vi "Process.vi"(8 "error in (no error)":errorcluster, 9 "Galvo.lvclass":refnum<class "Galvo.lvclass">, 10 "DAQ Class.lvclass":refnum<class "DAQ Class.lvclass">, 11 "Intensity Processing in":refnum<class "Intensity Processing.lvclass">) -> (0 "error out":errorcluster, 3 "Intensity Processing out":refnum<class "Intensity Processing.lvclass">)   [LabVIEW 2015, in "Intensity Processing.lvclass"]
uses:
  Intensity Processing.lvclass
  DAQ/DAQ Class.lvclass
  Galvo/Galvo.lvclass
  En Face States.ctl
  DAQ/DAQ Control Functional Global States.ctl
  Intensity Processing.lvclass/Intensity Processing.ctl
  <vilib>/Analysis/4window.llb/Hanning Window (DBL).vi
  <vilib>/Analysis/2dsp.llb/Real FFT.vi
  <vilib>/Analysis/4window.llb/AllCosWindow (DBL).vi
  Processing.lvclass
  Filter/Filter.lvclass
  <vilib>/Analysis/NI_AALPro.lvlib
panel:
  out "Stop Trim":dbl
  out "Start Trim":dbl
  out "Save Data":bool
  out "Save File Refnum":refnum<file>
  out "B-Scans Per Transfer":u32
  out "Points Per A-Scan":u32
  out "A-Scans Per B-Scan":u32
  out "Number of B-Scans":u32
  out "Background Noise":dbl[](array[numeric])
  out "Gain":dbl
  out "Log?":bool=TRUE
  out "Intensity Graph":sgl[][](graph)
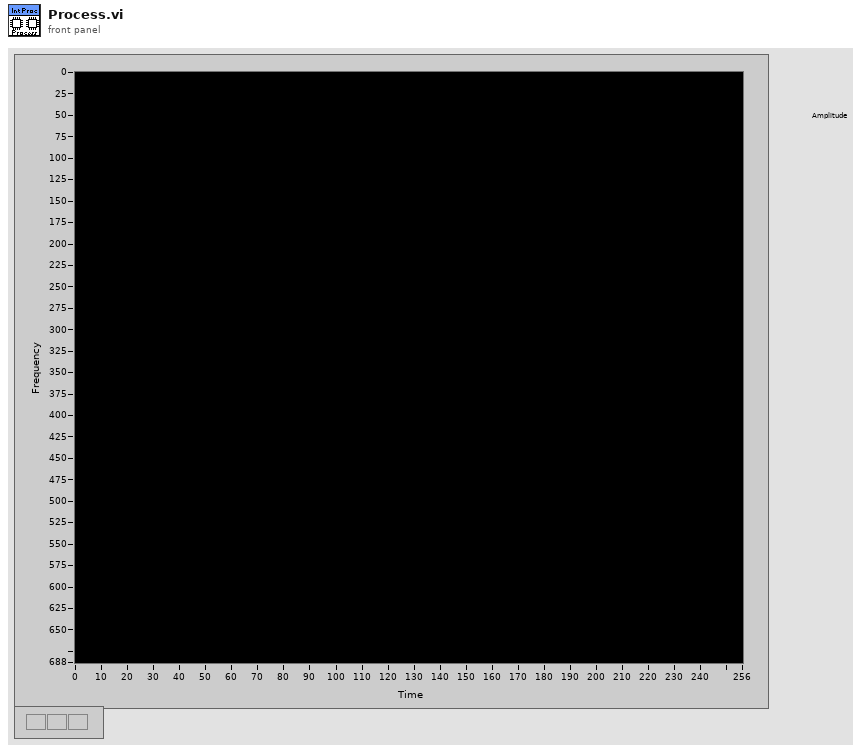
[diagram p1: front panel]
types:
  T1 = typedef "En Face States.ctl" = enum16{"Reset", "Update", "Get EnFace"}
  T2 = typedef "DAQ Class.lvclass/DAQ Parameters.ctl" = cluster{"Points Per A-Scan":u32, "A-Scans Per B-Scan":u32, "Number of B-Scans":u32, "B-Scans Per Transfer":u32, "Trigger Voltage":sgl, "Trigger Source":T3, "Trigger Slope":T4, "Channel":T5, "Clock":T6, "Bits per Sample":dbl, "Range":dbl, "Start Trim":u32, "Stop Trim":u32}
  T3 = typedef "DAQ Class.lvclass/Trigger Source.ctl" = enum16{"External", "Channel A", "Channel B"}
  T4 = typedef "DAQ Class.lvclass/Trigger Slope.ctl" = enum16{"Rising", "Falling"}
  T5 = typedef "OCT DAQ Channel Data Type.ctl" = enum16{"Channel 1", "Channel 2", "Channel 1 and 2"}
  T6 = typedef "DAQ Class.lvclass/Clock Control.ctl" = enum16{"Internal Clock", "External Clock"}
  T7 = enum16{"open", "replace", "create", "open or create", "replace or create", "replace or create with confirmation"}
  T8 = typedef "Galvo.lvclass/Scanning Cluster.ctl" = cluster{"Fast Axis Offset":sgl, "Slow Axis Offset":sgl, "Slow Axis Amp":sgl, "Fast Axis Amp":sgl, "Scan Pattern":enum16{"Raster", "Triangle Raster", "Sinusoid Raster"}}
  T9 = typedef "DAQ Control Functional Global States.ctl" = enum16{"Status", "Set Processing Finished", "Reset", "Clear", "Set DAQ Finished"}
  T10 = typedef "LVCursorListTypeDef.ctl" = cluster{"Name":string, "Color":u32, "Style":u8, "Point Style":u8, "Name Visible":bool, "Allow Drag":bool, "Cursor Mode":u32, "Plot":i32, "Index":i32, "Position":cluster{"X":dbl, "Y":dbl}, "X Scale":u32, "Y Scale":u32, "Watch Plots":i32[], "Watch All Plots":bool, "Plot Area":i32, "Label Offset":cluster{"X":dbl, "Y":dbl}}[]
  T11 = cluster{"Name":string, "Color":u32, "Style":u8, "Point Style":u8, "Name Visible":bool, "Allow Drag":bool, "Cursor Mode":u32, "Plot":i32, "Index":i32, "Position":cluster{"X":dbl, "Y":dbl}, "X Scale":u32, "Y Scale":u32, "Watch Plots":i32[], "Watch All Plots":bool, "Plot Area":i32, "Label Offset":cluster{"X":dbl, "Y":dbl}}
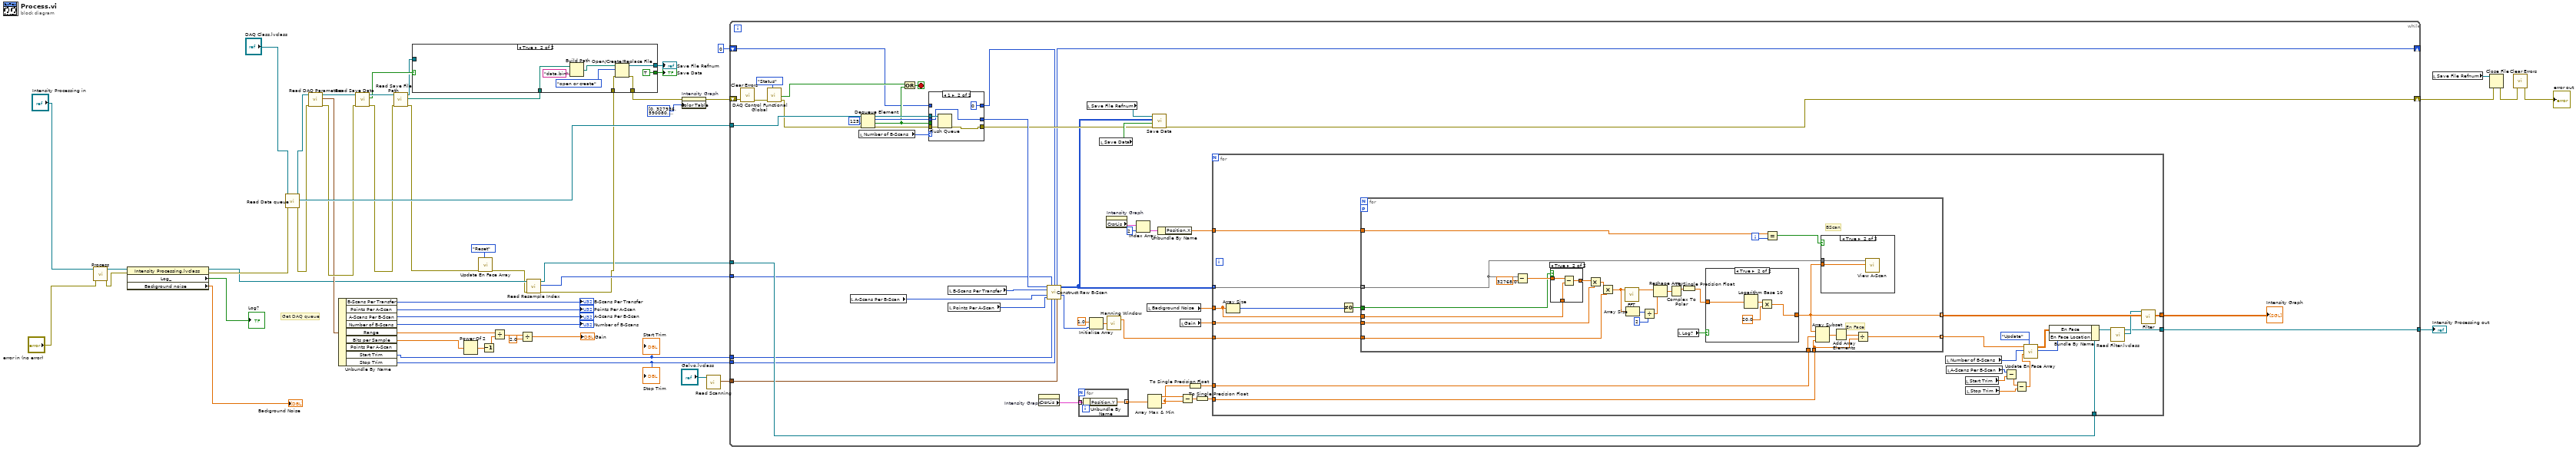
[diagram p0: block diagram]
diagram:
  # "Get DAQ queue"
  n1 = call-parent "Process.vi"("error in (no error)"="error in (no error)", "Processing in"="Intensity Processing in") -> ("error out"=w36:errorcluster, "Processing out"=w38:refnum<class "Intensity Processing.lvclass">)  [unwired: 8 in]
  n2 = property class="Intensity Processing.lvclass"(reference=w38, error in=w36) -> (reference out=w12:refnum<class "Intensity Processing.lvclass">, error out=w35:errorcluster, "Log_"=→"Log?":bool, "Background noise"=→"Background Noise":dbl[])
  n3 = call-dynamic "Read Data queue.vi"("error in (no error)"=w35, "DAQ Class in"="DAQ Class.lvclass") -> ("error out"=w50:errorcluster, "Data queue"=w51:refnum<queue>, "DAQ Class out"=w49:refnum<class "DAQ Class.lvclass">)  [unwired: 7 in]
  n4 = call-dynamic "Read DAQ Parameters.vi"("error in (no error)"=w50, "DAQ Class in"=w49) -> ("error out"=w32:errorcluster, "DAQ Parameters"=w26:T2, "DAQ Class out"=w34:refnum<class "DAQ Class.lvclass">)  [unwired: 7 in]
  n5 = Unbundle By Name(w26) -> ("B-Scans Per Transfer"=→"B-Scans Per Transfer":u32, "Points Per A-Scan"=→"Points Per A-Scan":u32, "A-Scans Per B-Scan"=→"A-Scans Per B-Scan":u32, "Number of B-Scans"=→"Number of B-Scans":u32, "Range"=w46:dbl, "Bits per Sample"=w47:dbl, "Start Trim"=w5:u32, "Stop Trim"=w6:u32)  [unwired: 1 out]
  "Start Trim" <- w5
  "Stop Trim" <- w6
  n6 = call-dynamic "Read Save Data.vi"("error in (no error)"=w32, "DAQ Class in"=w34) -> ("error out"=w33:errorcluster, "Save Data"=w30:bool, "DAQ Class out"=w31:refnum<class "DAQ Class.lvclass">)  [unwired: 7 in]
  n7 = call-dynamic "Read Save File Path.vi"("error in (no error)"=w33, "DAQ Class in"=w31) -> ("error out"=w17:errorcluster, "Save File Path"=w29:path, "DAQ Class out"=w25:refnum<class "DAQ Class.lvclass">)  [unwired: 7 in]
  n8 = Power Of 2(x=w47) -> (2^x=w48:dbl)
  n9 = call "Update En Face Array.vi"("State"=En_Face_States."Reset", "Error In"=w17) -> ("Error Out"=w9:errorcluster)  [unwired: 7 in, 2 out]
  n10 = Decrement(x=w48) -> (x-1=w45:dbl)
  n11 = Divide(x=w46, y=w45) -> (x/y=w24:dbl)
  n12 = Divide(x=w24, y=2.0) -> (x/y=→"Gain":dbl)
  n13 = call-dynamic "Read Resample Index.vi"("error in (no error)"=w9, "Processing in"=w12) -> ("error out"=w10:errorcluster, "Resample Index"=w11:i32[], "Processing out"=w8:refnum<class "Intensity Processing.lvclass">)  [unwired: 7 in]
  n14 = case shown="True" w30 {
    selector: w30 -> [w53 _]
    tunnel: w10 -> [w54 w62]
    tunnel: [w54 w61] -> w27
    tunnel: [_ w60] -> w15
    tunnel: [w53 TRUE] -> w14
    tunnel: w29 -> [_ w58]
    tunnel: w25 -> [_ _]
    frame False {
    }
    frame True {
      n15 = Build Path(base path=w58, name or relative path="data.bin") -> (appended path=w57:path)
      n16 = Open/Create/Replace File(file path (use dialog)=w57, error in=w62, operation (0:open)=T7."open or create") -> (refnum out=w60:refnum<file>, error out=w61:errorcluster)  [unwired: 3 in, 1 out]
    }
  }
  "Save File Refnum" <- w15
  "Save Data" <- w14
  n17 = property on="Intensity Graph" class="IntGraph (strict)"(error in=w27, "Color Table"=u32[] [0, 327936, 590080, 852224, 983296, 1114624, 1180160, 1311232, 1442304, 1573632, 1704704, 1770240, 1901312, 1966848, 2098176, 2163712, 2294784, 2491392, 2557184, 2688256, 2753792, 2884864, 2950656, 3081728, 3147264, 3344129, 3475457, 3540993, 3672321, 3738113, 3869185, 3934977, 4066305, 4197633, 4328961, 4394497, 4460289, 4591617, 4657409, 4788481, 4854273, 4985601, 5116929, 5248257, 5314049, 5379841, 5511169, 5576961, 5708033, 5773825, 5905153, 6036482, 6167810, 6233346, 6299138, 6430466, 6496258, 6562050, 6693634, 6759426, 6890754, 7022082, 7087874, 7153666, 7284994, 7350786, 7482114, 7547906, 7613698, 7745026, 7876354, 8007682, 8073474, 8139522, 8205314, 8336642, 8467970, 8533763, 8599555, 8665347, 8731139, 8862467, 8993795, 9059587, 9125380, 9191428, 9257220, 9388548, 9454340, 9520132, 9585924, 9717253, 9848837, 9914629, 9980165, 10045957, 10177541, 10243334, 10309126, 10375174, 10440966, 10572294, 10703623, 10769416, 10835208, 10901256, 10967049, 11033097, 11033609, 11099401, 11165450, 11231242, 11231754, 11297547, 11363339, 11429131, 11495180, 11495692, 11561740, 11693069, 11758861, 11759373, 11825165, 11891214, 11957006, 12022799, 12023311, 12089103, 12220944, 12286736, 12286736, 12352529, 12418577, 12484370, 12550162, 12615954, 12681747, 12747796, 12813588, 12813845, 12879894, 12945686, 13077015, 13142808, 13143064, 13208856, 13274905, 13340697, 13340953, 13472282, 13538075, 13604379, 13670172, 13735964, 13801757, 13867550, 13933343, 13999392, 13999648, 14065441, 14131234, 14197027, 14197541, 14263334, 14329383, 14395176, 14460969, 14592553, 14658346, 14724139, 14789932, 14790189, 14856238, 14922287, 14988080, 15053873, 15054130, 15119923, 15185972, 15251765, 15317559, 15383353, 15449146, 15449660, 15515454, 15515968, 15516226, 15582021, 15582278, 15582536, 15648587, 15648844, 15714639, 15714897, 15715155, 15780949, 15781463, 15847256, 15847770, 15848028, 15913823, 15914081, 15979875, 15980133, 15980391, 16046441, 16046444, 16046703, 16046705, 16112500, 16113015, 16113274, 16113277, 16179072, 16179330, 16179588, 16245384, 16245387, 16245389, 16245648, 16311443, 16376982, 16377241, 16377499, 16443294, 16443553, 16443555, 16443815, 16509866, 16510124, 16510127, 16575923, 16575924, 16576182, 16576441, 16576443, 16576702, 16576705, 16576963, 16577222, 16577224, 16577482, 16577485, 16577743, 16577745, 16578004, 16578262, 16578264, 16578523, 16578782, 16579040, 16579299, 16579301, 16579303, 16579562, 16579821]) -> (error out=w28:errorcluster)  [unwired: 1 in, 1 out]
  n18 = call-dynamic "Read Scanning.vi"("Galvo in"="Galvo.lvclass") -> ("Scanning Parameters"=w3:T8)  [unwired: 8 in, 2 out]
  n19 = while {
    tunnel: w51 -> [w101]
    shift-right: [w79] -> w43
    shift-left: w28 -> [w111]
    tunnel: w11 -> [w67]
    tunnel: w8 -> [w71]
    shift-right: [w70] -> _
    shift-left: 0 -> [w69]
    tunnel: w6 -> [w66]
    tunnel: w5 -> [w65]
    tunnel: w3 -> [w64]
    tunnel: [w63] -> w1
    stop <- w104 stop-if-true
    n20 = call <vilib>:"Clear Errors.vi"("error in (no error)"=w111) -> ("error out"=w110:errorcluster)  [unwired: 5 in, 1 out]
    n21 = call "DAQ Control Functional Global.vi"("State"=DAQ_Control_Functional_Global_States."Status", "Error In"=w110) -> ("Error Out"=w100:errorcluster, "Reset?"=w102:bool)  [unwired: 6 in, 2 out]
    n22 = local read "A-Scans Per B-Scan"() -> (w85:u32)
    n23 = local read "Number of B-Scans"() -> (w86:u32)
    n24 = Dequeue Element(queue=w101, timeout in ms (-1)=125, error in (no error)=w100) -> (queue out=w97:refnum<queue>, element=w98:u16[], timed out?=w94:bool, error out=w96:errorcluster)
    n25 = Or(x=w102, y=w94) -> (x .or. y?=w104:bool)
    n26 = case shown="1" w86 {
      tunnel: w98 -> [w177 w179]
      tunnel: w97 -> [_ w181]
      tunnel: [w177 w179] -> w89
      tunnel: w94 -> [_ _]
      tunnel: w96 -> [w176 w182]
      tunnel: [w176 w180] -> w80
      tunnel: w69 -> [w175 _]
      tunnel: [w175 u32 0 ("B-Scan Processed Out")] -> w68
      frame 0, Default {
      }
      frame 1 {
        n27 = Flush Queue(queue=w181, error in (no error)=w182) -> (error out=w180:errorcluster)  [unwired: 2 out]
      }
    }
    n28 = local read "B-Scans Per Transfer"() -> (w84:u32)
    n29 = local read "Points Per A-Scan"() -> (w83:u32)
    n30 = property on="Intensity Graph" class="IntGraph (strict)"() -> ("CrsrLis"=w106:T10)  [unwired: 2 in, 2 out]
    n31 = call "Construct Raw B-Scan.vi"("1D Raw Data In"=w89, "Resample Array"=w67, "B-Scan Processed In"=w68, "B-Scans Per Transfer"=w84, "A-Scans Per B-Scan"=w85, "Points Per A-Scan"=w83, "Start Trim"=w65, "Stop Trim"=w66, "Scanning Parameters"=w64) -> ("B-Scan Processed Out"=w70:u32, "B-Scan In"=w78:u16[][][], "A-Scan Size"=w74:i32)  [unwired: 4 in]
    n32 = for {
      tunnel: w106 -> [w184] mode=indexing
      tunnel: [w183] -> w105 mode=indexing
      n33 = Unbundle By Name(w184) -> ("Position.Y"=w183:dbl)
    }
    n34 = local read "Save File Refnum"() -> (w82:refnum<file>)
    n35 = Initialize Array(1.0 ("element"), w74) -> (w76:dbl[])
    n36 = local read "Save Data"() -> (w81:bool)
    n37 = property on="Intensity Graph" class="IntGraph (strict)"() -> ("CrsrLis"=w93:T10)  [unwired: 2 in, 2 out]
    n38 = call-poly <vilib>:"Hanning Window.vi"("X"=w76) -> ("Windowed X"=w75:dbl[])  [unwired: 1 out]
    n39 = Index Array(array=w93, index=2) -> (element=w91:T11)
    n40 = local read "Background Noise"() -> (w88:dbl[])
    n41 = Array Max & Min(array=w105) -> (max value=w109:dbl, min value=w107:dbl)  [unwired: 2 out]
    n42 = call "Save Data.vi"("error in (no error)"=w80, ">> Save Data? >>"=w81, "U16 Array"=w78, "Byte Stream File in"=w82) -> ("error out"=w79:errorcluster)  [unwired: 7 in]
    n43 = Unbundle By Name(w91) -> ("Position.X"=w90:dbl)
    n44 = local read "Gain"() -> (w87:dbl)
    n45 = Subtract(x=w109, y=w107) -> (x-y=w108:dbl)
    n46 = To Single Precision Float(number=w107) -> (single precision float=w72:sgl)
    n47 = To Single Precision Float(number=w108) -> (single precision float=w73:sgl)
    n48 = for {
      tunnel: w73 -> [w136]
      tunnel: w72 -> [w135]
      tunnel: w87 -> [w134]
      tunnel: [w125] -> w95
      tunnel: w90 -> [w131]
      tunnel: w78 -> [w122] mode=indexing
      tunnel: w88 -> [w130]
      tunnel: w75 -> [w129]
      tunnel: w71 -> [w116]
      tunnel: [w112] -> w63
      n49 = Array Size(array=w130) -> (size(s)=w133:i32)
      n50 = Not Equal To 0?(x=w133) -> (x != 0?=w132:bool)
      n51 = for {
        tunnel: w129 -> [w163]
        tunnel: [w139] -> w124 mode=indexing
        tunnel: w136 -> [w158]
        tunnel: w135 -> [w161]
        tunnel: [w138] -> w126 mode=indexing
        tunnel: w134 -> [w156]
        tunnel: w122 -> [w137] mode=indexing
        tunnel: w130 -> [w148]
        tunnel: w132 -> [w146]
        workers-P: _ -> [_]
        tunnel: w131 -> [w144]
        i -> [w145]
        # "BScan"
        # "En Face"
        n52 = Subtract(x=w137, y=32768.0) -> (x-y=w149:dbl[])
        n53 = case shown="True" w146 {
          tunnel: w149 -> [w166 w169]
          tunnel: w148 -> [_ w168]
          tunnel: [w166 w167] -> w147
          frame False {
          }
          frame True {
            n54 = Subtract(x=w169, y=w168) -> (x-y=w167:dbl[])
          }
        }
        n55 = Multiply(x=w147, y=w156) -> (x*y=w150:dbl[])
        n56 = Multiply(x=w150, y=w163) -> (x*y=w152:dbl[])
        n57 = call-poly <vilib>:"FFT.vi"("X"=w152) -> ("FFT {X}"=w162:cdb[])  [unwired: 9 in, 1 out]
        n58 = Array Size(array=w152) -> (size(s)=w155:i32)
        n59 = Divide(x=w155, y=2) -> (x/y=w153:dbl)
        n60 = Reshape Array(w162, w153) -> (w142:cdb[])
        n61 = Complex To Polar(r * e^(i*theta)=w142) -> (r=w141:dbl[])  [unwired: 1 out]
        n62 = local read "Log?"() -> (w157:bool)
        n63 = To Single Precision Float(number=w141) -> (single precision float=w140:sgl[])
        n64 = case shown="True" w157 {
          tunnel: w140 -> [w170 w174]
          tunnel: [w170 w171] -> w139
          frame False {
          }
          frame True {
            n65 = Logarithm Base 10(1:w174) -> (0:w173:sgl[])
            n66 = Multiply(x=w173, y=sgl 20.0 ("element")) -> (x*y=w171:sgl[])
          }
        }
        n67 = Equal?(x=w144, y=w145) -> (x = y?=w143:bool)
        n68 = Array Subset(array=w139, index=w161, length=w158) -> (w160:sgl[])
        n69 = case shown="True" w143 {
          tunnel: w137 -> [_ w165]
          tunnel: w139 -> [_ w164]
          frame False {
          }
          frame True {
            n70 = call "View A-Scan.vi"("A-Scan Processed"=w164, "A-Scan (Raw)"=w165) -> ()  [unwired: 10 in]
          }
        }
        n71 = Add Array Elements(numeric array=w160) -> (sum=w159:sgl)
        n72 = Divide(x=w159, y=w158) -> (x/y=w138:sgl)
      }
      n73 = local read "Number of B-Scans"() -> (w128:u32)
      n74 = local read "A-Scans Per B-Scan"() -> (w121:u32)
      n75 = local read "Start Trim"() -> (w120:dbl)
      n76 = local read "Stop Trim"() -> (w118:dbl)
      n77 = Subtract(x=w121, y=w120) -> (x-y=w119:dbl)
      n78 = Subtract(x=w119, y=w118) -> (x-y=w117:dbl)
      n79 = call "Update En Face Array.vi"("State"=En_Face_States."Update", "A-Scans Per B-Scan"=w117, "Number Of BScans"=w128, "Slice"=w126) -> ("B-Scan Index"=w113:i32, "Array out"=w115:sgl[][])  [unwired: 5 in, 1 out]
      n80 = Bundle By Name(cluster=w116, "En Face"=w115, "En Face Location"=w113) -> (w114:refnum<class "Intensity Processing.lvclass">)
      n81 = call-dynamic "Read Filter.lvclass.vi"("Processing in"=w114) -> ("Filter.lvclass"=w123:refnum<class "Filter.lvclass">, "Processing out"=w112:refnum<class "Intensity Processing.lvclass">)  [unwired: 8 in, 1 out]
      n82 = call-dynamic "Filter.vi"("Input"=w124, "Filter in"=w123) -> ("Output"=w125:sgl[][])  [unwired: 7 in, 2 out]
    }
    "Intensity Graph" <- w95
  }
  "Intensity Processing out" <- w1
  n83 = local read "Save File Refnum"() -> (w13:refnum<file>)
  n84 = Close File(refnum=w13, error in=w43) -> (error out=w40:errorcluster)  [unwired: 1 out]
  n85 = call <vilib>:"Clear Errors.vi"("error in (no error)"=w40) -> ("error out"=→"error out":errorcluster)  [unwired: 5 in, 1 out]
